vi "PlanVirtualStave - Copy.vi"(7 "Stave Locking Points [mm]":dbl[][](array[numeric])=[[0.0, 0.0, 0.0], [280.05, 0.0, 0.0], [574.05, 0.0, 0.0], [868.05, 0.0, 0.0], [1162.05, 0.0, 0.0]], 8 "Working height [mm]":dbl, 10 "Module fiducial marker":T3(ring), 11 "Tape Type":enum16{"Stereo", "Axial"}(ring)=enum."Axial") -> (0 "Module fiducials in the Stave's basis":T1(graph)=[{"Generated List of Module Coordinates"=[-7.69, 87.79, 87.79, -7.69, 90.31, 185.79000000000002, 185.79000000000002, 90.31, 188.31, 283.79, 283.79, 188.31, 286.31, 381.79, 381.79, 286.31, 384.31, 479.79, 479.79, 384.31, 482.31, 577.79, 577.79, 482.31, 580.31, 675.79, 675.79, 580.31, 678.31, 773.79, 773.79, 678.31, 776.31, 871.79, 871.79, 776.31, 874.31, 969.79, 969.79, 874.31, 972.31, 1067.79, 1067.79, 972.31, 1070.31, 1165.79, 1165.79, 1070.31, 1168.31, 1263.79, 1263.79, 1168.31], "Generated List of Module Coordinates"=[-16.132, -16.132, -113.21200000000002, -113.21200000000002, -16.132, -16.132, -113.21200000000002, -113.21200000000002, -16.132, -16.132, -113.21200000000002, -113.21200000000002, -16.132, -16.132, -113.21200000000002, -113.21200000000002, -16.132, -16.132, -113.21200000000002, -113.21200000000002, -16.132, -16.132, -113.21200000000002, -113.21200000000002, -16.132, -16.132, -113.21200000000002, -113.21200000000002, -16.132, -16.132, -113.21200000000002, -113.21200000000002, -16.132, -16.132, -113.21200000000002, -113.21200000000002, -16.132, -16.132, -113.21200000000002, -113.21200000000002, -16.132, -16.132, -113.21200000000002, -113.21200000000002, -16.132, -16.132, -113.21200000000002, -113.21200000000002, -16.132, -16.132, -113.21200000000002, -113.21200000000002]}, {"Generated List of Module Coordinates"=[0.0, 280.05, 574.05, 868.05, 1162.05], "Generated List of Module Coordinates"=[0.0, 0.0, 0.0, 0.0, 0.0]}], 3 "Generated List: Coordinates of Fiducials on Modules":dbl[][](array[numeric])=[[-7.69, -16.132, 0.0], [87.79, -16.132, 0.0], [87.79, -113.21200000000002, 0.0], [-7.69, -113.21200000000002, 0.0], [90.31, -16.132, 0.0], [185.79000000000002, -16.132, 0.0], [185.79000000000002, -113.21200000000002, 0.0], [90.31, -113.21200000000002, 0.0], [188.31, -16.132, 0.0], [283.79, -16.132, 0.0], [283.79, -113.21200000000002, 0.0], [188.31, -113.21200000000002, 0.0], [286.31, -16.132, 0.0], [381.79, -16.132, 0.0], [381.79, -113.21200000000002, 0.0], [286.31, -113.21200000000002, 0.0], [384.31, -16.132, 0.0], [479.79, -16.132, 0.0], [479.79, -113.21200000000002, 0.0], [384.31, -113.21200000000002, 0.0], [482.31, -16.132, 0.0], [577.79, -16.132, 0.0], [577.79, -113.21200000000002, 0.0], [482.31, -113.21200000000002, 0.0], [580.31, -16.132, 0.0], [675.79, -16.132, 0.0], [675.79, -113.21200000000002, 0.0], [580.31, -113.21200000000002, 0.0], [678.31, -16.132, 0.0], [773.79, -16.132, 0.0], [773.79, -113.21200000000002, 0.0], [678.31, -113.21200000000002, 0.0], [776.31, -16.132, 0.0], [871.79, -16.132, 0.0], [871.79, -113.21200000000002, 0.0], [776.31, -113.21200000000002, 0.0], [874.31, -16.132, 0.0], [969.79, -16.132, 0.0], [969.79, -113.21200000000002, 0.0], [874.31, -113.21200000000002, 0.0], [972.31, -16.132, 0.0], [1067.79, -16.132, 0.0], [1067.79, -113.21200000000002, 0.0], [972.31, -113.21200000000002, 0.0], [1070.31, -16.132, 0.0], [1165.79, -16.132, 0.0], [1165.79, -113.21200000000002, 0.0], [1070.31, -113.21200000000002, 0.0], [1168.31, -16.132, 0.0], [1263.79, -16.132, 0.0], [1263.79, -113.21200000000002, 0.0], [1168.31, -113.21200000000002, 0.0]])   [LabVIEW 2016]
panel:
  out "output cluster":cluster{dbl[], dbl[]}
  out "Y centreline":dbl
  in  "Module centre [mm]":T2
  in  "N modules":dbl=13.0
  in  "Module width [mm]":dbl=97.54
  in  "Module pitch [mm]":dbl=98.0
  # "Based on Sutcliffe Drawings:\n\nDistance to EOS, axial = [ -7.69, -16.132 ]\nstereo = [ -9.591, 115.081 ]"
  # "Provided by Camera Calibration:"
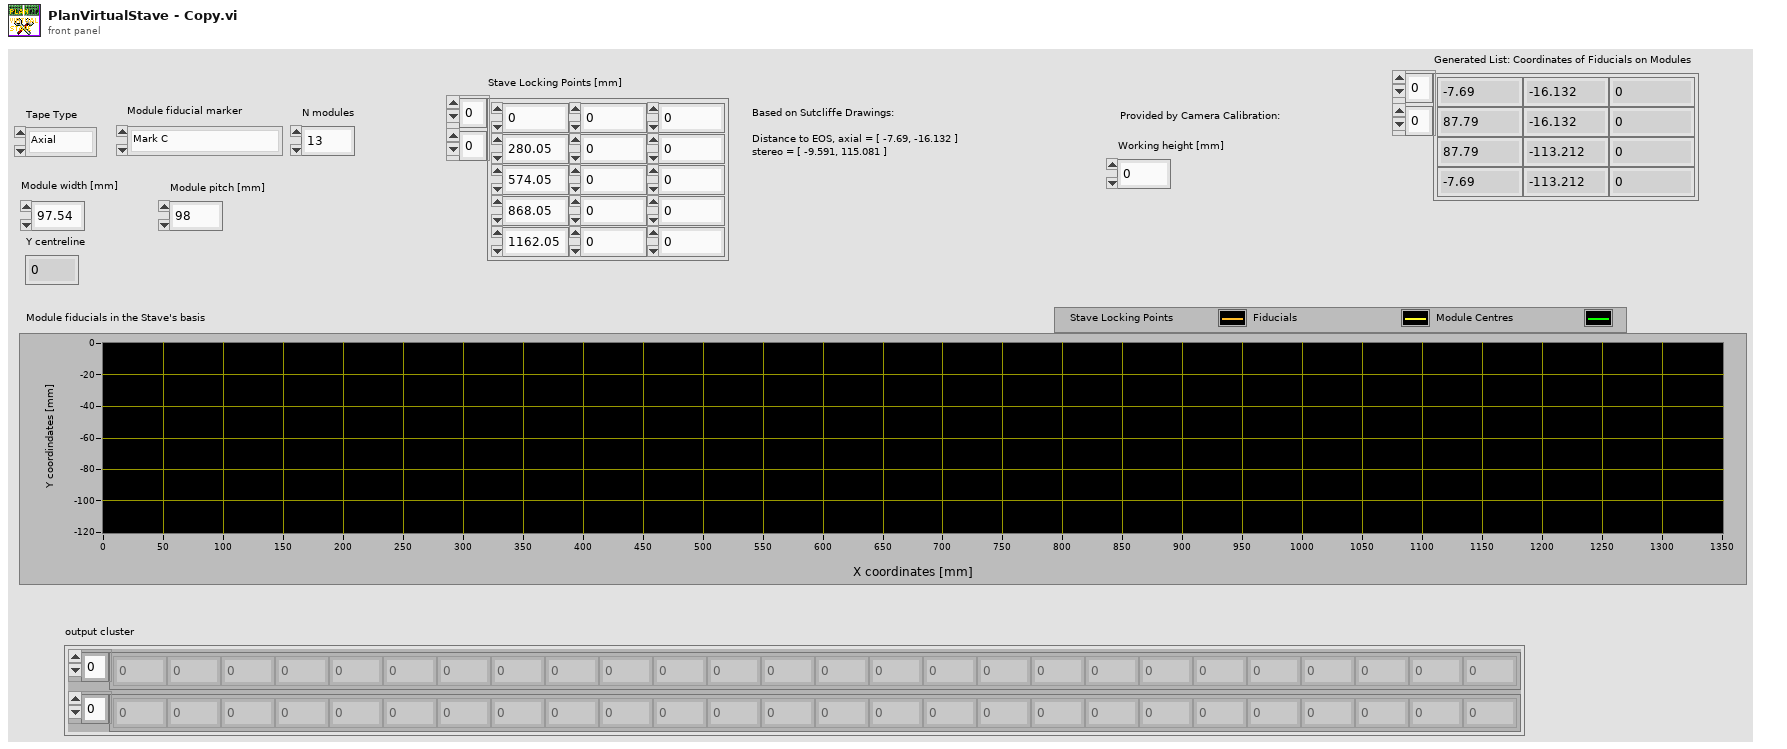
[diagram p1: front panel]
types:
  T1 = cluster{"Generated List of Module Coordinates":dbl[], "Generated List of Module Coordinates":dbl[]}[]
  T2 = cluster{"X [mm]":dbl, "Y [mm]":dbl, "Z [mm]":dbl}
  T3 = enum16{"Mark C", "Mark B", "Strip Corner", "[None]"}
  T4 = cluster{"Generated List of Module Coordinates":dbl[], "Generated List of Module Coordinates":dbl[]}
  T5 = cluster{"Stave Locking Points [mm]":dbl[], "Stave Locking Points [mm]":dbl[]}
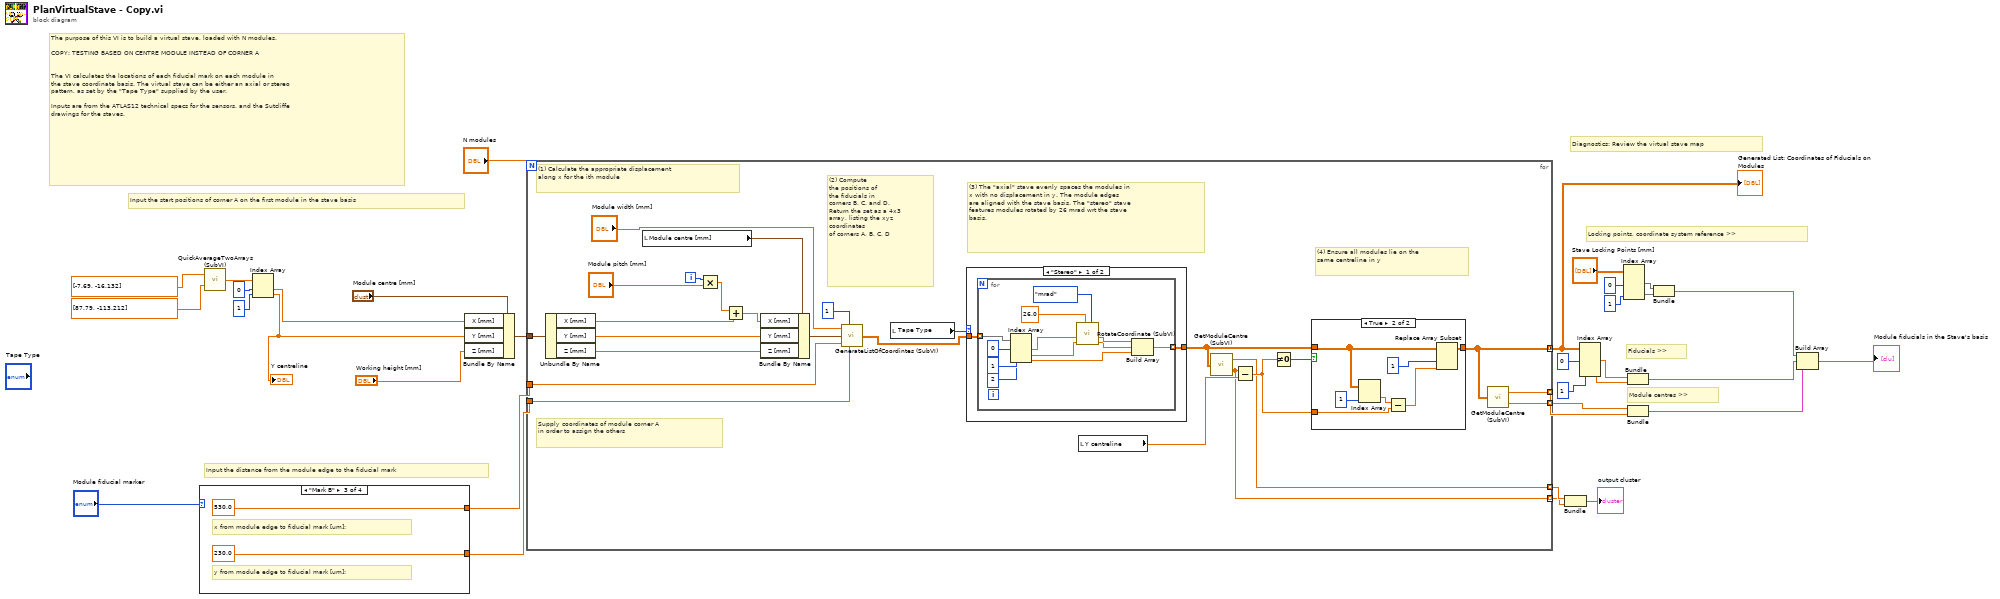
[diagram p0: block diagram]
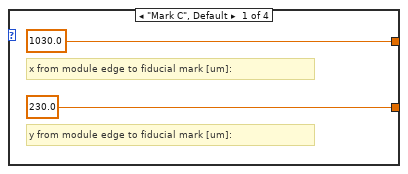
[diagram p4: hidden frame]
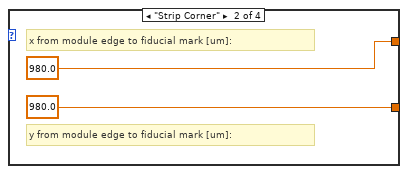
[diagram p5: hidden frame]
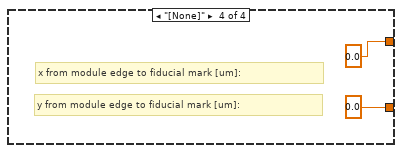
[diagram p6: hidden frame]
diagram:
  # "Locking points, coordinate system reference >>"
  # "Module centres >>"
  # "Fiducials >>"
  # "Diagnostics: Review the virtual stave map"
  # "Input the start positions of corner A on the first module in the stave basis"
  # "Input the distance from the module edge to the fiducial mark"
  # "The purpose of this VI is to build a virtual stave, loaded with N modules.\n\nCOPY: TESTING BASED ON CENTRE MODULE INSTEAD OF CORNER A\n\n\nThe VI calculates the locations of each fiducial mark on each module in \nthe stave coordinate basis. The virtual stave can be either an axial or stereo \npattern, as set by the \"Tape Type\" supplied by the user.\n\nInputs are from the ATLAS12 technical specs for the sensors, and the Sutcliffe\ndrawings for the staves."
  n1 = case shown="\"Mark B\"" "Module fiducial marker" {
    tunnel: [1030.0 980.0 530.0 0.0] -> w32
    tunnel: [230.0 980.0 230.0 0.0] -> w31
    frame "Mark C", Default {
      # "y from module edge to fiducial mark [um]:"
      # "x from module edge to fiducial mark [um]:"
    }
    frame "Strip Corner" {
      # "y from module edge to fiducial mark [um]:"
      # "x from module edge to fiducial mark [um]:"
    }
    frame "Mark B" {
      # "y from module edge to fiducial mark [um]:"
      # "x from module edge to fiducial mark [um]:"
    }
    frame "[None]" {
      # "y from module edge to fiducial mark [um]:"
      # "x from module edge to fiducial mark [um]:"
    }
  }
  n2 = call "QuickAverageTwoArrays (SubVI).vi"("B"=dbl[] [87.79, -113.212], "A"=dbl[] [-7.69, -16.132]) -> ("Average of A and B"=w6:dbl[])
  n3 = Index Array(array=w6, index #1=0 ("index"), index #2=1 ("index")) -> (element #1=w3:dbl, element #2=w1:dbl)
  "Y centreline" <- w1
  n4 = Bundle By Name(cluster="Module centre [mm]", "X [mm]"=w3, "Y [mm]"=w1, "Z [mm]"="Working height [mm]") -> (w25:T2)
  n5 = for {
    N: "N modules" -> [_]
    tunnel: w32 -> [w55]
    tunnel: w31 -> [w65]
    tunnel: w25 -> [w54]
    tunnel: [w47] -> w19 mode=concatenating
    tunnel: [w46] -> w16 mode=indexing
    tunnel: [w45] -> w15 mode=indexing
    tunnel: [w43] -> w10 mode=indexing
    tunnel: [w42] -> w9 mode=indexing
    i -> [w64]
    # "(4) Ensure all modules lie on the \nsame centreline in y"
    # "(3) The \"axial\" stave evenly spaces the modules in \nx with no displacement in y. The module edges \nare aligned with the stave basis. The \"stereo\" stave \nfeatures modules rotated by 26 mrad wrt the stave\nbasis."
    # "(2) Compute\nthe positions of \nthe fiducials in \ncorners B, C, and D. \nReturn the set as a 4x3\narray, listing the xyz \ncoordinates\nof corners A, B, C, D"
    # "(1) Calculate the appropriate displacement \nalong x for the ith module"
    # "Supply coordinates of module corner A \nin order to assign the others"
    n6 = Unbundle By Name(w54) -> ("X [mm]"=w63:dbl, "Y [mm]"=w61:dbl, "Z [mm]"=w59:dbl)
    n7 = local read "Module centre [mm]"() -> (w57:T2)
    n8 = Multiply(x=w64, y="Module pitch [mm]") -> (x*y=w62:dbl)
    n9 = Add(x=w62, y=w63) -> (x+y=w60:dbl)
    n10 = Bundle By Name(cluster=w57, "X [mm]"=w60, "Y [mm]"=w61, "Z [mm]"=w59) -> (w58:T2)
    n11 = call "GenerateListOfCoordintes (SubVI).vi"("Module side length [mm]"="Module width [mm]", "Nloops"=1, "A [mm]"=w58, "x to fiducial [um]"=w55, "y to fiducial [um]"=w65) -> ("Generated List of Module Coordinates"=w51:dbl[][])  [unwired: 4 in]
    n12 = local read "Tape Type"() -> (w53:enum16{"Stereo", "Axial"})
    n13 = case shown="\"Stereo\"" w53 {
      tunnel: [w76 w89] -> w49
      tunnel: w51 -> [w75 w89]
      frame "Stereo" {
        n14 = for {
          tunnel: [w78] -> w76 mode=indexing
          tunnel: w75 -> [w77] mode=indexing
          n15 = Index Array(array=w77, index #1=0 ("index"), index #2=1 ("index"), index #3=2 ("index")) -> (element #1=w83:dbl, element #2=w82:dbl, element #3=w79:dbl)
          n16 = call "RotateCoordinate (SubVI).vi"("Units"=enum16{"mrad", "Radians", "Degrees"}."mrad", "Angle"=26.0, "y"=w82, "x"=w83) -> ("y'"=w80:dbl, "x'"=w81:dbl)  [unwired: 6 in]
          n17 = Build Array(w81, w80, w79) -> (w78:dbl[])
        }
      }
      frame "Axial", Default {
      }
    }
    n18 = local read "Y centreline"() -> (w52:dbl)
    n19 = call "GetModuleCentre (SubVI).vi"("4x3 Array of Fiducial Coordinates"=w49) -> ("x, centre"=w43:dbl, "y, centre"=w42:dbl)
    n20 = Subtract(x=w42, y=w52) -> (x-y=w48:dbl)
    n21 = Not Equal To 0?(x=w48) -> (x != 0?=w50:bool)
    n22 = case shown="True" w50 {
      tunnel: w49 -> [w67 w74]
      tunnel: w48 -> [_ w69]
      tunnel: [w67 w68] -> w47
      frame False {
      }
      frame True {
        n23 = Index Array(array=w74, index (col)=1 ("disabled index (col)")) -> (element=w72:dbl[])  [unwired: 1 in]
        n24 = Subtract(x=w72, y=w69) -> (x-y=w71:dbl[])
        n25 = Replace Array Subset(array=w74, new element=w71, index (col)=1 ("disabled index (col)")) -> (w68:dbl[][])  [unwired: 1 in]
      }
    }
    n26 = call "GetModuleCentre (SubVI).vi"("4x3 Array of Fiducial Coordinates"=w47) -> ("x, centre"=w46:dbl, "y, centre"=w45:dbl)
  }
  "Generated List: Coordinates of Fiducials on Modules" <- w19
  n27 = Bundle(w10, w9) -> (→"output cluster":cluster{dbl[], dbl[]})  [unwired: 1 in]
  n28 = Index Array(array=w19, index (col) #1=0 ("disabled index (col)"), index (col) #2=1 ("index (col)")) -> (element #1=w30:dbl[], element #2=w29:dbl[])  [unwired: 2 in]
  n29 = Index Array(array="Stave Locking Points [mm]", index (col) #1=0 ("disabled index (col)"), index (col) #2=1 ("disabled index (col)")) -> (element #1=w21:dbl[], element #2=w20:dbl[])  [unwired: 2 in]
  n30 = Bundle("Generated List of Module Coordinates"=w30, "Generated List of Module Coordinates"=w29) -> (w14:T4)  [unwired: 1 in]
  n31 = Bundle(w16, w15) -> (w13:cluster{dbl[], dbl[]})  [unwired: 1 in]
  n32 = Bundle("Stave Locking Points [mm]"=w21, "Stave Locking Points [mm]"=w20) -> (w12:T5)  [unwired: 1 in]
  n33 = Build Array(w12, w14, w13) -> (→"Module fiducials in the Stave's basis":T1)
